vi "Sin LUT.vi"() -> ()   [LabVIEW 2015]
doc: "This VI demonstrates the functionality of a look-up table (LUT) using the sbRIO. It references a predefined table in the Sin LUT (subVI).vi to index values corresponding to a sine waveform. It then outputs the waveform on the eight LEDs of the evaluation board.\n\nThe potentiometer can be used to very the frequency of the sine wave output."
uses:
  <vilib>/rvi/Emulation/niFpgaGetClockAttributes.vi
  <vilib>/rvi/Emulation/niFpgaSctlEmulationGetInTimedLoop.vi
  <vilib>/rvi/Emulation/niFpgaEmulationReportErrorSimple.vi
  <vilib>/rvi/Emulation/niFpgaCriticalErrorInLSC.vi
panel:
  in  "stop":bool
  # "This VI demonstrates the functionality of a look-up table (LUT) on the eval kit FPGA. It references a predefined table in the Sin LUT (subVI).vi to index values corresponding to a sine waveform.  It then outputs the waveform on the eight LEDs of the evaluation board.\n\nThe potentiometer can be used to vary the frequency of the sine wave output."
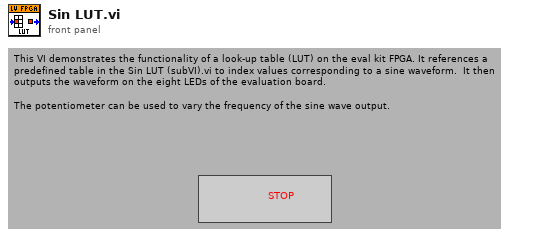
[diagram p1: front panel]
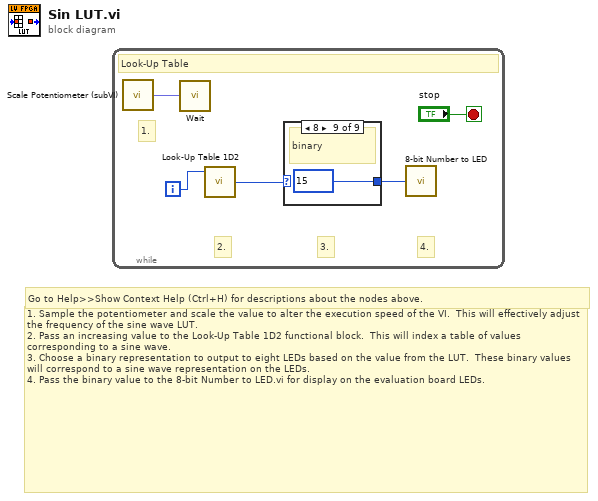
[diagram p0: block diagram]
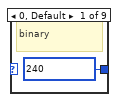
[diagram p2: hidden frame]
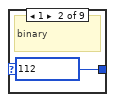
[diagram p3: hidden frame]
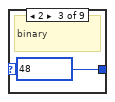
[diagram p4: hidden frame]
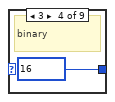
[diagram p5: hidden frame]
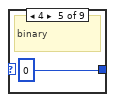
[diagram p6: hidden frame]
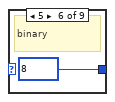
[diagram p7: hidden frame]
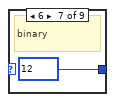
[diagram p8: hidden frame]
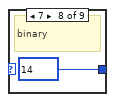
[diagram p9: hidden frame]
diagram:
  # "Go to Help>>Show Context Help (Ctrl+H) for descriptions about the nodes above."
  # "1. Sample the potentiometer and scale the value to alter the execution speed of the VI.  This will effectively adjust the frequency of the sine wave LUT.\n2. Pass an increasing value to the Look-Up Table 1D2 functional block.  This will index a table of values corresponding to a sine wave.\n3. Choose a binary representation to output to eight LEDs based on the value from the LUT.  These binary values will correspond to a sine wave representation on the LEDs.\n4. Pass the binary value to the 8-bit Number to LED.vi for display on the evaluation board LEDs."
  n1 = while {
    i -> [w3]
    stop <- "stop" stop-if-true
    # "4."
    # "3."
    # "2."
    # "1."
    # "Look-Up Table"
    n2 = call "Scale Potentiometer (subVI).vi"() -> ("Wait (us)"=w1:fxp<+/-,42,21>)  [unwired: 1 out]
    n3 = call "Wait"("Count(uSec)"=w1) -> ()  [unwired: 1 out]
    n4 = call "Look-Up Table 1D2"("address"=w3) -> ("data out"=w2:i16)  [unwired: 8 in]
    n5 = case shown="8" w2 {
      tunnel: [u8 240 u8 112 u8 48 u8 16 u8 0 u8 8 u8 12 u8 14 u8 15] -> w4
      frame 0, Default {
        # "binary"
      }
      frame 1 {
        # "binary"
      }
      frame 2 {
        # "binary"
      }
      frame 3 {
        # "binary"
      }
      frame 4 {
        # "binary"
      }
      frame 5 {
        # "binary"
      }
      frame 6 {
        # "binary"
      }
      frame 7 {
        # "binary"
      }
      frame 8 {
        # "binary"
      }
    }
    n6 = call "8-bit Number to LED.vi"("6-bit Unsigned\n Number (0-63)"=w4) -> ()  [unwired: 1 out]
  }
